vi "Close File.vi"(8 "error in (no error)":errorcluster, 9 "Perform Post Actions?":bool, 10 "File Post Action":refnum<class "File Post Action.lvclass">[](array[class]), 11 "File Writer in":refnum<class "File Writer.lvclass">) -> (0 "error out":errorcluster, 3 "File Writer out":refnum<class "File Writer.lvclass">)   [LabVIEW 2020, in "File Writer.lvlib" / "File Writer.lvclass"]
doc: "Close the file and then perform File Post Actions if requested."
uses:
  File Writer.lvclass
  File Post Action/File Post Action.lvclass
  File Writer.lvclass/File Writer.ctl
  <vilib>/Utility/file.llb/Is Path and Not Empty.vi
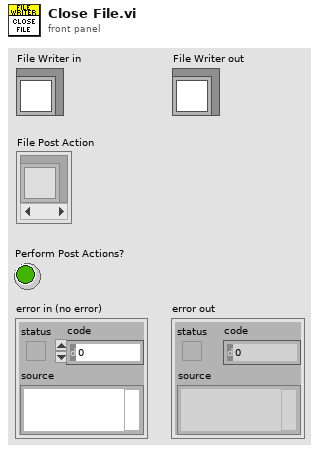
[diagram p1: front panel]
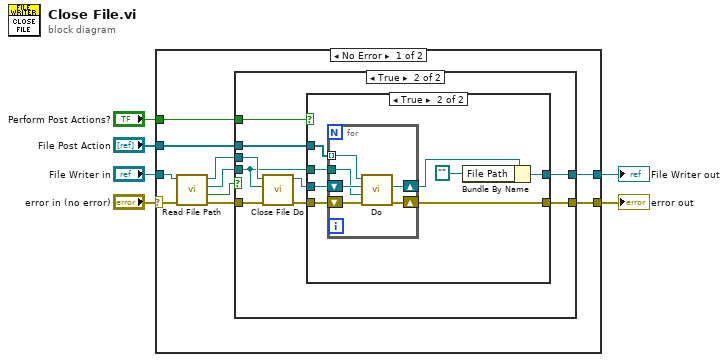
[diagram p0: block diagram]
diagram:
  n1 = case shown="No Error" "error in (no error)" {
    selector: "error in (no error)" -> [w7 w45]
    tunnel: [w15 w45] -> w5
    tunnel: [w16 w44] -> w3
    tunnel: "File Writer in" -> [w12 w44]
    tunnel: "Perform Post Actions?" -> [w13 _]
    tunnel: "File Post Action" -> [w14 _]
    frame No Error {
      n2 = call "Read File Path.vi"("error in (no error)"=w7, "File Writer in"=w12) -> ("error out"=w8:errorcluster, "Is Active?"=w11:bool, "File Path"=w10:path, "File Writer out"=w9:refnum<class "File Writer.lvclass">)  [unwired: 6 in]
      n3 = case shown="True" w11 {
        tunnel: [w18 w26] -> w16
        tunnel: w9 -> [w18 w23]
        tunnel: [w17 w27] -> w15
        tunnel: w8 -> [w17 w21]
        tunnel: w14 -> [_ w25]
        tunnel: w13 -> [_ w24]
        tunnel: w10 -> [_ w19]
        frame False {
        }
        frame True {
          n4 = call-dynamic "Close File Do.vi"("error in (no error)"=w21, "File Path"=w19, "File Writer in"=w23) -> ("error out"=w20:errorcluster, "File Writer out"=w22:refnum<class "File Writer.lvclass">)  [unwired: 7 in]
          n5 = case shown="True" w24 {
            tunnel: w22 -> [w29 w37]
            tunnel: w20 -> [w28 w36]
            tunnel: [w28 w35] -> w27
            tunnel: [w29 w31] -> w26
            tunnel: w25 -> [_ w33]
            tunnel: w19 -> [_ w32]
            frame False {
            }
            frame True {
              n6 = for {
                shift-right: [w40] -> w34
                shift-left: w37 -> [w43]
                shift-right: [w39] -> w35
                shift-left: w36 -> [w41]
                tunnel: w33 -> [w42] mode=indexing
                tunnel: w32 -> [w38]
                n7 = call-dynamic "Do.vi"("error in (no error)"=w41, "File Path"=w38, "File Writer in"=w43, "File Post Action in"=w42) -> ("error out"=w39:errorcluster, "File Writer out"=w40:refnum<class "File Writer.lvclass">)  [unwired: 6 in]
              }
              n8 = Bundle By Name(cluster=w34, "File Path"=path "") -> (w31:refnum<class "File Writer.lvclass">)
            }
          }
        }
      }
    }
    frame Error {
    }
  }
  "error out" <- w5
  "File Writer out" <- w3
